vi "Define USIM SUCI Key Pair.vi"(7 "Private Key (\"A0\")":string="A0", 8 "error in (no error)":errorcluster, 9 "Public Key (\"A0\")":string="A0", 10 "SIM Profile (\"SIM1\")":string="SIM1", 11 "VISA resource name":refnum<visa-resource-name>) -> (0 "error out":errorcluster, 3 "VISA resource name out":refnum<visa-resource-name>)   [LabVIEW 2015, in "Rohde&Schwarz CMXP Base.lvlib"]
doc: "Specifies the subscription concealed identifier (SUCI) as a pair of the home network public key identifier and the home network private key. The home network private key is entered as a 64-digit hexadecimal number.\n\nAttribute:\n-\n\nRemote-control command:\n[CONFigure:]SIMProfile:USIM:SECurity:HNPPkpair"
uses:
  <instrlib>/Rohde&Schwarz CMXP Base/Rohde&Schwarz CMXP Base.lvlib
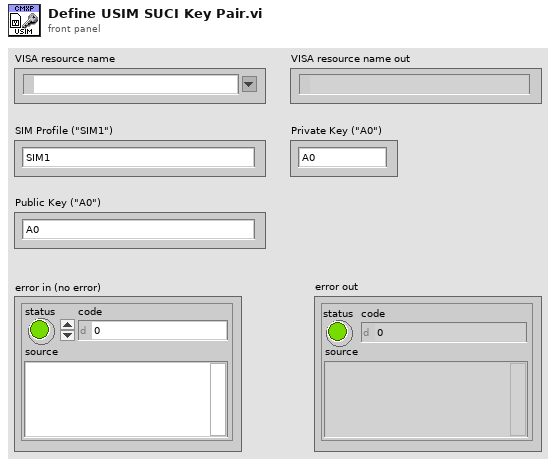
[diagram p1: front panel]
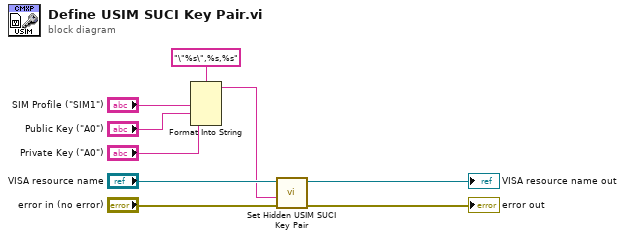
[diagram p0: block diagram]
diagram:
  n1 = Format Into String(format string="\"%s\",%s,%s", "SIM Profile (\"SIM1\")", "Public Key (\"A0\")", "Private Key (\"A0\")") -> (resulting string=w1:string)  [unwired: 2 in, 1 out]
  n2 = call "Set Hidden USIM SUCI Key Pair"("error in (no error)"="error in (no error)", "Hidden USIM SUCI Key Pair ()"=w1, "instrument handle"="VISA resource name") -> ("error out"=→"error out":errorcluster, "instrument handle out"=→"VISA resource name out":refnum<visa-resource-name>)  [unwired: 7 in]
